vi "全局 水样时间.vi"() -> ()   [LabVIEW 2016]
panel:
  in  "选择发送的参数":string
  in  "time20":string
  in  "time19":string
  in  "time18":string
  in  "time17":string
  in  "time16":string
  in  "time15":string
  in  "time14":string
  in  "time13":string
  in  "time12":string
  in  "time11":string
  in  "time10":string
  in  "time9":string
  in  "time8":string
  in  "time7":string
  in  "time6":string
  in  "time5":string
  in  "time4":string
  in  "time3":string
  in  "time2":string
  in  "time1":string
  in  "小时数据时间":string
  in  "时间":string
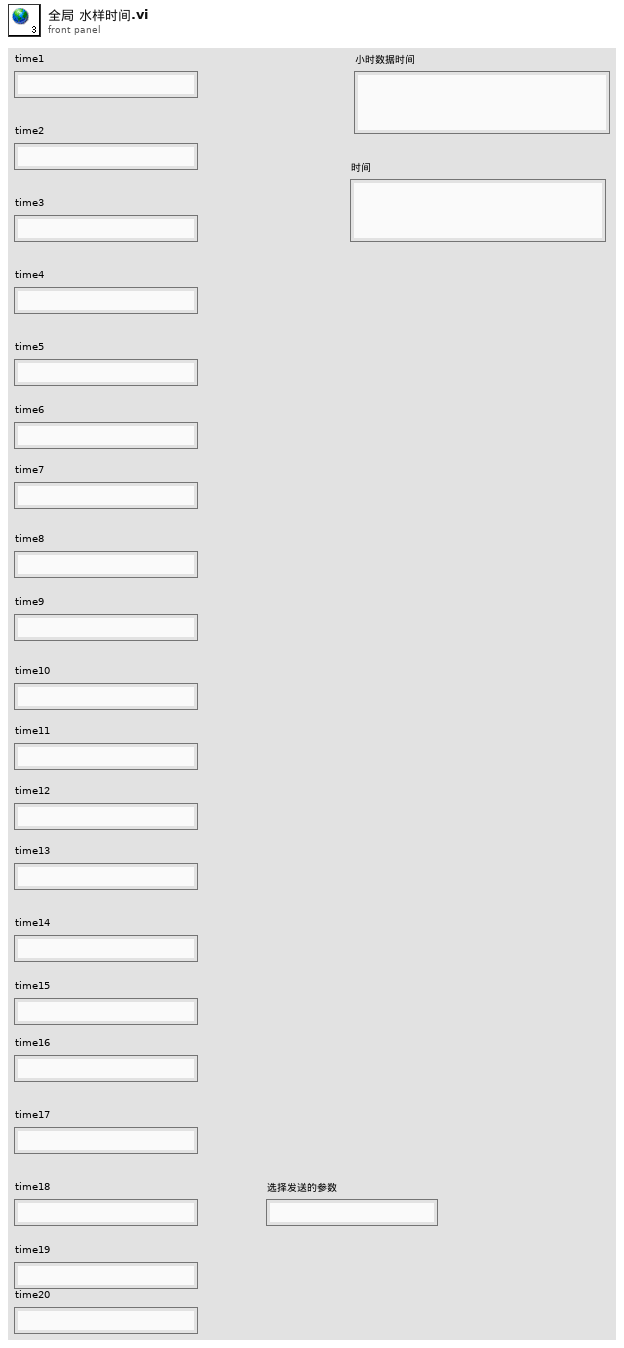
[diagram p1: front panel]
diagram:
